vi "editscenario load fields and operations.vi"(8 "error in (no error)":errorcluster, 9 "Template Keys (empty)":T1, 11 "Connection Refnum":T2) -> (0 "error out":errorcluster, 1 "Template Keys":T1, 3 "Connection Refnum":T2)   [LabVIEW 2011]
uses:
  SI.LIB/ODBC/SQL Controls/Connection Refnum.ctl
  Addons/internet/utils/keyedarr.llb/Keyed Array.ctl
  server/database/Users/User Record Fields.ctl
  server/database/Fields/Field DataTypes.ctl
  server/database/Stations/Station Record Fields.ctl
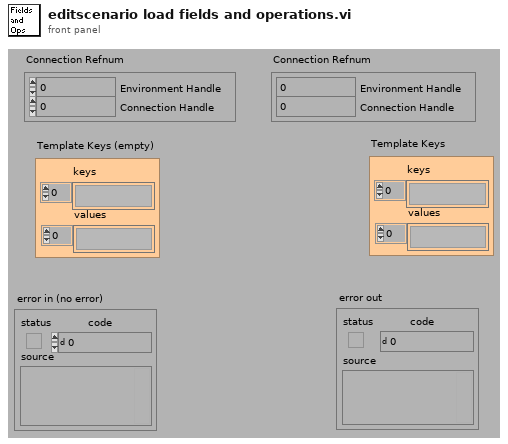
[diagram p1: front panel]
types:
  T1 = typedef "Keyed Array.ctl" = cluster{"keys":string[], "values":string[]}
  T2 = typedef "Connection Refnum.ctl" = cluster{"Environment Handle":i32, "Connection Handle":i32}
  T3 = typedef "Field Record.ctl" = cluster{"ixField":i32, "iSequenceOrder":i32, "sxFieldId":string, "sxSequenceId":string, "sDisplayName":string, "sValue":string, "sUnits":string, "nDataType":T4, "nNextItem":T5, "fSystem":bool, "fSystemValue":bool, "fRequired":bool, "fSetAtTest":bool, "fTestField":bool, "fDeleted":bool, "fIndexed":bool, "fFreeList":bool}
  T4 = typedef "Field DataTypes.ctl" = enum32{"text", "numeric", "list", "timestamp", "boolean"}
  T5 = typedef "Field NextItem.ctl" = enum32{"Reset", "Retain", "Auto-Increment"}
  T6 = typedef "User Record Fields.ctl" = enum32{"sxUsername", "sLastName", "sFirstName", "sEmail", "sPassword", "tLoginTime", "sLoginComputer", "fAdministrator", "fRunSequences", "fModifySequences", "fRunScenarios", "fModifyScenarios", "fModifyTemplates", "fModifyUsers", "fModifyStations", "fModifyFields", "ixUser"}
  T7 = typedef "Station Record Fields.ctl" = enum32{"sxStationId", "sIP", "fVerified", "ixStation"}
  T8 = typedef "User Record.ctl" = cluster{"ixUser":i32, "sxUsername":string, "sLastName":string, "sFirstName":string, "sEmail":string, "sPassword":string, "tLoginTime":timestamp, "sLoginComputer":string, "fAdministrator":bool, "fRunSequences":bool, "fModifySequences":bool, "fRunScenarios":bool, "fModifyScenarios":bool, "fModifyTemplates":bool, "fModifyUsers":bool, "fModifyStations":bool, "fModifyFields":bool}
  T9 = typedef "Sequence Record.ctl" = cluster{"ixSequence":i32, "sxSequenceId":string, "sDescription":string, "sCreator":string, "tCreationDate":timestamp, "sModifier":string, "tModifiedDate":timestamp, "fApproved":bool, "fSpartanSetsSN":bool, "fOverwriteData":bool, "fStopOnFail":bool, "fDisableQuickMode":bool, "fPartialExecution":bool, "fAutoNextItem":bool, "fDoNotPrintOnFail":bool}
  T10 = typedef "Station Record.ctl" = cluster{"ixStation":i32, "sxStationId":string, "sIP":string, "fVerified":bool}
  T11 = typedef "Test Record.ctl" = cluster{"ixTest":i32, "sxTestId":string, "sVersion":string, "sDriverTypes":string[], "sDescription":string, "iQuickMode":i32}
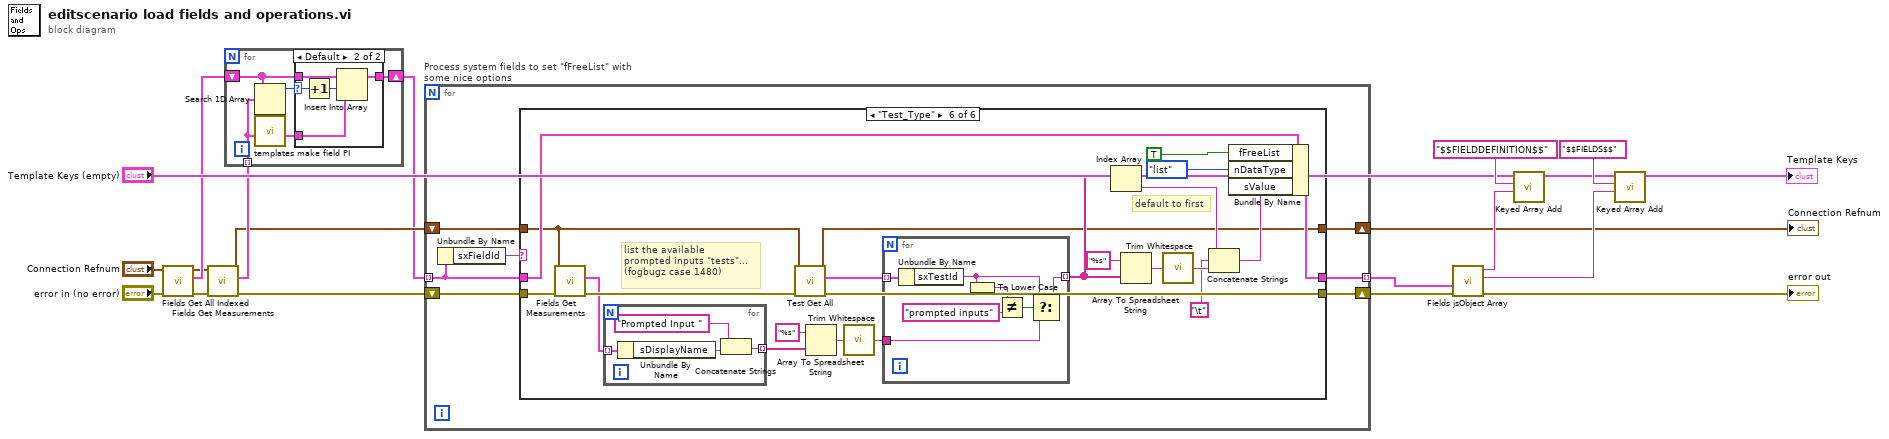
[diagram p0: block diagram]
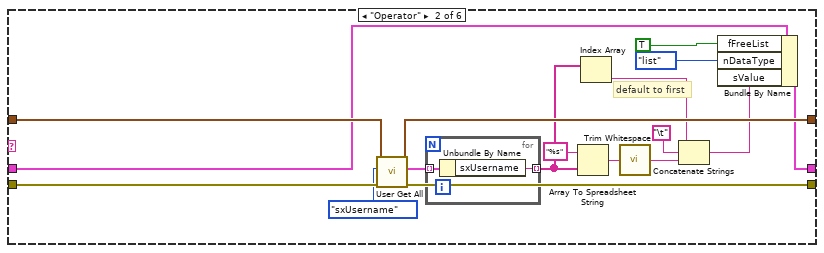
[diagram p4: hidden frame]
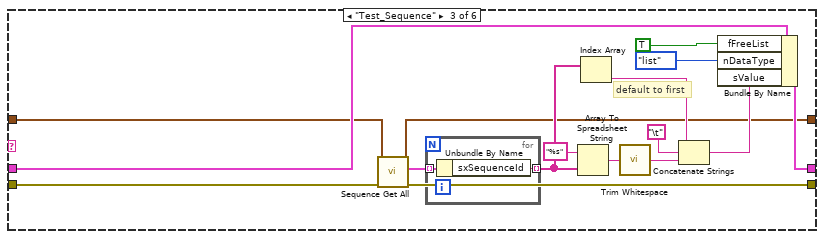
[diagram p5: hidden frame]
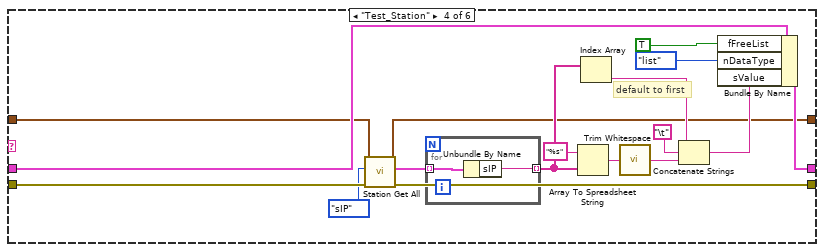
[diagram p6: hidden frame]
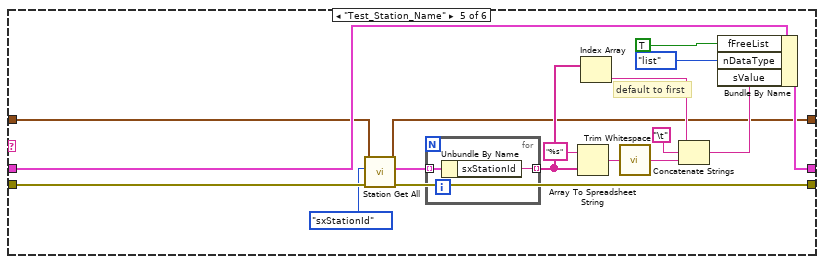
[diagram p7: hidden frame]
diagram:
  n1 = call "Fields Get All Indexed.vi"("error in (no error)"="error in (no error)", "Connection Refnum"="Connection Refnum") -> ("error out"=w6:errorcluster, "Fields Out"=w8:T3[], "Connection Refnum"=w7:T2)  [unwired: 7 in]
  n2 = call "Fields Get Measurements.vi"("error in (no error)"=w6, "Connection Refnum"=w7) -> ("error out"=w4:errorcluster, "Measurement Fields"=w9:T3[], "dup Connection Refnum"=w2:T2)  [unwired: 1 in, 6 out]
  n3 = for {
    shift-right: [w24] -> w1
    shift-left: w8 -> [w25]
    tunnel: w9 -> [w21] mode=indexing
    n4 = Search 1D Array(1D array=w25, element=w21) -> (index of element=w22:i32)  [unwired: 1 out]
    n5 = call "templates make field PI.vi"("Field Information  2"=w21) -> ("Field Information"=w23:T3)  [unwired: 10 out]
    n6 = case shown="Default" w22 {
      selector: w22 -> [_ w27]
      tunnel: w25 -> [w26 w31]
      tunnel: [w26 w30] -> w24
      tunnel: w23 -> [_ w29]
      frame -1 {
      }
      frame Default {
        n7 = Increment(x=w27) -> (x+1=w28:i32)
        n8 = Insert Into Array(array=w31, index=w28, new element=w29) -> (w30:T3[])
      }
    }
  }
  n9 = for "Process system fields to set \"fFreeList\" with some nice options" {
    tunnel: w1 -> [w38] mode=indexing
    tunnel: [w37] -> w11 mode=indexing
    shift-right: [w32] -> w13
    shift-left: w4 -> [w35]
    shift-right: [w33] -> w12
    shift-left: w2 -> [w34]
    n10 = Unbundle By Name(w38) -> ("sxFieldId"=w36:string)
    n11 = case shown="\"Test_Type\"" w36 {
      tunnel: w38 -> [w41 w54 w76 w95 w114 w138]
      tunnel: [w41 w53 w75 w94 w113 w137] -> w37
      tunnel: w35 -> [w39 w58 w66 w83 w102 w122]
      tunnel: w34 -> [w40 w57 w64 w85 w104 w117]
      tunnel: [w40 w55 w63 w84 w103 w127] -> w33
      tunnel: [w39 w56 w65 w82 w101 w128] -> w32
      frame "NOP", Default {
      }
      frame "Operator" {
        # "default to first"
        n12 = call "User Get All.vi"("error in (no error)"=w58, "Sort by Field (sxUsername)"=User_Record_Fields."sxUsername" ("Sort by Field (Username)"), "Connection Refnum"=w57) -> ("error out"=w56:errorcluster, "User Records"=w50:T8[], "Connection Refnum"=w55:T2)  [unwired: 1 in, 5 out]
        n13 = for {
          tunnel: w50 -> [w60] mode=indexing
          tunnel: [w59] -> w44 mode=indexing
          n14 = Unbundle By Name(w60) -> ("sxUsername"=w59:string)
        }
        n15 = Array To Spreadsheet String(array=w44, 3:"%s") -> (spreadsheet string=w47:string)  [unwired: 1 out]
        n16 = Index Array(array=w44) -> (element=w43:string)  [unwired: 1 in]
        n17 = call <vilib>:"Trim Whitespace.vi"("string"=w47) -> ("trimmed string"=w46:string)  [unwired: 1 in]
        n18 = Concatenate Strings(w43, "\t", w46) -> (w45:string)
        n19 = Bundle By Name(cluster=w54, "fFreeList"=TRUE, "nDataType"=Field_DataTypes."list", "sValue"=w45) -> (w53:T3)
      }
      frame "Test_Sequence" {
        # "default to first"
        n20 = call "Sequence Get All.vi"("error in (no error)"=w66, "Connection Refnum"=w64) -> ("error out"=w65:errorcluster, "Sequence Records"=w62:T9[], "Connection Refnum"=w63:T2)  [unwired: 2 in, 5 out]
        n21 = for {
          tunnel: [w78] -> w68 mode=indexing
          tunnel: w62 -> [w77] mode=indexing
          n22 = Unbundle By Name(w77) -> ("sxSequenceId"=w78:string)
        }
        n23 = Array To Spreadsheet String(array=w68, 3:"%s") -> (spreadsheet string=w71:string)  [unwired: 1 out]
        n24 = Index Array(array=w68) -> (element=w67:string)  [unwired: 1 in]
        n25 = call <vilib>:"Trim Whitespace.vi"("string"=w71) -> ("trimmed string"=w70:string)  [unwired: 1 in]
        n26 = Concatenate Strings(w67, "\t", w70) -> (w69:string)
        n27 = Bundle By Name(cluster=w76, "fFreeList"=TRUE, "nDataType"=Field_DataTypes."list", "sValue"=w69) -> (w75:T3)
      }
      frame "Test_Station" {
        # "default to first"
        n28 = call "Station Get All.vi"("error in (no error)"=w83, "Sort by (sxStationId)"=Station_Record_Fields."sIP" ("Sort by (TestStation_ID)"), "Connection Refnum"=w85) -> ("error out"=w82:errorcluster, "Station Records"=w81:T10[], "Connection Refnum"=w84:T2)  [unwired: 1 in, 5 out]
        n29 = for {
          tunnel: [w97] -> w87 mode=indexing
          tunnel: w81 -> [w96] mode=indexing
          n30 = Unbundle By Name(w96) -> ("sIP"=w97:string)
        }
        n31 = Array To Spreadsheet String(array=w87, 3:"%s") -> (spreadsheet string=w90:string)  [unwired: 1 out]
        n32 = Index Array(array=w87) -> (element=w86:string)  [unwired: 1 in]
        n33 = call <vilib>:"Trim Whitespace.vi"("string"=w90) -> ("trimmed string"=w89:string)  [unwired: 1 in]
        n34 = Concatenate Strings(w86, "\t", w89) -> (w88:string)
        n35 = Bundle By Name(cluster=w95, "fFreeList"=TRUE, "nDataType"=Field_DataTypes."list", "sValue"=w88) -> (w94:T3)
      }
      frame "Test_Station_Name" {
        # "default to first"
        n36 = call "Station Get All.vi"("error in (no error)"=w102, "Sort by (sxStationId)"=Station_Record_Fields."sxStationId" ("Sort by (TestStation_ID)"), "Connection Refnum"=w104) -> ("error out"=w101:errorcluster, "Station Records"=w100:T10[], "Connection Refnum"=w103:T2)  [unwired: 1 in, 5 out]
        n37 = for {
          tunnel: [w116] -> w106 mode=indexing
          tunnel: w100 -> [w115] mode=indexing
          n38 = Unbundle By Name(w115) -> ("sxStationId"=w116:string)
        }
        n39 = Array To Spreadsheet String(array=w106, 3:"%s") -> (spreadsheet string=w109:string)  [unwired: 1 out]
        n40 = Index Array(array=w106) -> (element=w105:string)  [unwired: 1 in]
        n41 = call <vilib>:"Trim Whitespace.vi"("string"=w109) -> ("trimmed string"=w108:string)  [unwired: 1 in]
        n42 = Concatenate Strings(w105, "\t", w108) -> (w107:string)
        n43 = Bundle By Name(cluster=w114, "fFreeList"=TRUE, "nDataType"=Field_DataTypes."list", "sValue"=w107) -> (w113:T3)
      }
      frame "Test_Type" {
        # "list the available\nprompted inputs \"tests\"...\n(fogbugz case 1480)"
        # "default to first"
        n44 = call "Fields Get Measurements.vi"("error in (no error)"=w122, "Connection Refnum"=w117) -> ("error out"=w121:errorcluster, "Measurement Fields"=w120:T3[])  [unwired: 1 in, 7 out]
        n45 = for {
          tunnel: w120 -> [w142] mode=indexing
          tunnel: [w139] -> w119 mode=indexing
          n46 = Unbundle By Name(w142) -> ("sDisplayName"=w140:string)
          n47 = Concatenate Strings("Prompted Input " ("y"), w140) -> (w139:string)
        }
        n48 = call "Test Get All.vi"("error in (no error)"=w121, "Connection Refnum"=w117) -> ("error out"=w128:errorcluster, "Test Records"=w126:T11[], "Connection Refnum"=w127:T2)  [unwired: 2 in, 5 out]
        n49 = Array To Spreadsheet String(array=w119, 3:"%s") -> (spreadsheet string=w125:string)  [unwired: 1 out]
        n50 = call <vilib>:"Trim Whitespace.vi"("string"=w125) -> ("trimmed string"=w123:string)  [unwired: 1 in]
        n51 = for {
          tunnel: w126 -> [w149] mode=indexing
          tunnel: [w144] -> w130 mode=indexing
          tunnel: w123 -> [w143]
          n52 = Unbundle By Name(w149) -> ("sxTestId"=w145:string)
          n53 = To Lower Case(string=w145) -> (all lower case string=w147:string)
          n54 = Not Equal?(x=w147, y="prompted inputs") -> (x != y?=w146:bool)
          n55 = Select(t=w145, s=w146, f=w143) -> (s? t:f=w144:string)
        }
        n56 = Index Array(array=w130) -> (element=w129:string)  [unwired: 1 in]
        n57 = Array To Spreadsheet String(array=w130, 3:"%s") -> (spreadsheet string=w133:string)  [unwired: 1 out]
        n58 = call <vilib>:"Trim Whitespace.vi"("string"=w133) -> ("trimmed string"=w132:string)  [unwired: 1 in]
        n59 = Concatenate Strings(w129, "\t", w132) -> (w131:string)
        n60 = Bundle By Name(cluster=w138, "fFreeList"=TRUE, "nDataType"=Field_DataTypes."list", "sValue"=w131) -> (w137:T3)
      }
    }
  }
  "Connection Refnum" <- w12
  n61 = call "Fields jsObject Array.vi"("error in (no error)"=w13, "FIELDS (none)"=w11) -> ("error out"=→"error out":errorcluster, "Fields jsObject Array"=w16:string, "Field jsObject Definition"=w17:string)  [unwired: 2 in, 5 out]
  n62 = call "Keyed Array Add.vi"("value"=w17, "key"="$$FIELDDEFINITION$$", "array in"="Template Keys (empty)") -> ("array out"=w18:T1)  [unwired: 1 in, 3 out]
  n63 = call "Keyed Array Add.vi"("value"=w16, "key"="$$FIELDS$$", "array in"=w18) -> ("array out"=→"Template Keys":T1)  [unwired: 1 in, 3 out]
